vi "GET_Series.vi"(6 "get all issues":bool=TRUE, 7 "progress ref":refnum<vi>, 8 "error in (no error)":errorcluster, 10 "series URL":string, 11 "ComicVine_class in":refnum<class "series_class.lvclass">) -> (0 "error out":errorcluster, 3 "ComicVine_class out":refnum<class "series_class.lvclass">)   [LabVIEW 2024, in "series_class.lvclass"]
uses:
  series_class.lvclass
  series_class.lvclass/series_class.ctl
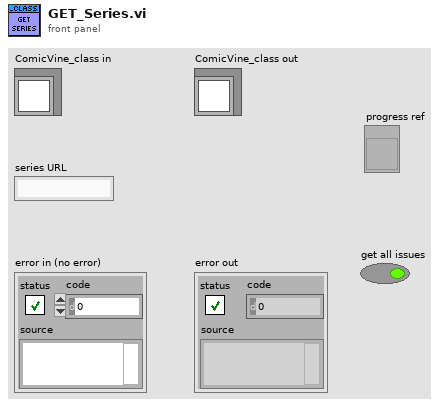
[diagram p1: front panel]
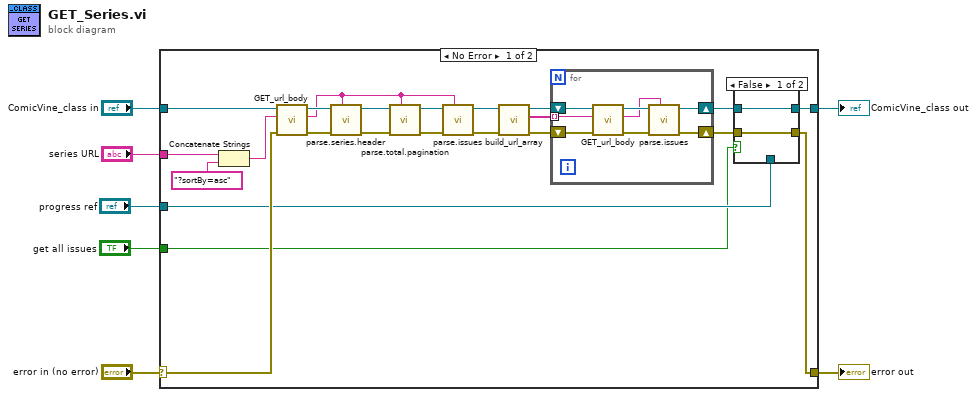
[diagram p0: block diagram]
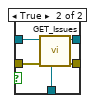
[diagram p2: hidden frame]
diagram:
  n1 = case shown="No Error" "error in (no error)" {
    selector: "error in (no error)" -> [w28 w47]
    tunnel: [w11 w47] -> w6
    tunnel: [w13 w46] -> w4
    tunnel: "ComicVine_class in" -> [w30 w46]
    tunnel: "series URL" -> [w23 _]
    tunnel: "progress ref" -> [w9 _]
    tunnel: "get all issues" -> [w8 _]
    frame No Error {
      n2 = Concatenate Strings(w23, "?sortBy=asc") -> (w22:string)
      n3 = call-dynamic "GET_url_body.vi"("error in (no error)"=w28, "url"=w22, "comic_class in"=w30) -> ("error out"=w27:errorcluster, "body"=w15:string, "comic_class out"=w29:refnum<class "series_class.lvclass">)  [unwired: 6 in]
      n4 = call "parse.series.header.vi"("series body"=w15, "error in (no error)"=w27, "ComicVine_class in"=w29) -> ("error out"=w25:errorcluster, "ComicVine_class out"=w26:refnum<class "series_class.lvclass">)  [unwired: 7 in]
      n5 = call "parse.total.pagination.vi"("series body"=w15, "error in (no error)"=w25, "ComicVine_class in"=w26) -> ("error out"=w10:errorcluster, "ComicVine_class out"=w21:refnum<class "series_class.lvclass">)  [unwired: 6 in, 1 out]
      n6 = call "parse.issues.vi"("series body"=w15, "error in (no error)"=w10, "ComicVine_class in"=w21) -> ("error out"=w19:errorcluster, "ComicVine_class out"=w20:refnum<class "series_class.lvclass">)  [unwired: 7 in]
      n7 = call "build_url_array.vi"("error in (no error)"=w19, "ComicVine_class in"=w20) -> ("error out"=w18:errorcluster, "urls"=w16:string[], "ComicVine_class out"=w17:refnum<class "series_class.lvclass">)  [unwired: 7 in]
      n8 = for {
        shift-right: [w39] -> w12
        shift-left: w18 -> [w42]
        shift-right: [w45] -> w14
        shift-left: w17 -> [w41]
        tunnel: w16 -> [w40] mode=indexing
        n9 = call-dynamic "GET_url_body.vi"("error in (no error)"=w42, "url"=w40, "comic_class in"=w41) -> ("error out"=w44:errorcluster, "body"=w38:string, "comic_class out"=w43:refnum<class "series_class.lvclass">)  [unwired: 6 in]
        n10 = call "parse.issues.vi"("series body"=w38, "error in (no error)"=w44, "ComicVine_class in"=w43) -> ("error out"=w39:errorcluster, "ComicVine_class out"=w45:refnum<class "series_class.lvclass">)  [unwired: 7 in]
      }
      n11 = case shown="False" w8 {
        tunnel: w14 -> [w31 w37]
        tunnel: [w31 w36] -> w13
        tunnel: w12 -> [w32 w35]
        tunnel: [w32 w34] -> w11
        tunnel: w9 -> [_ w33]
        frame False {
        }
        frame True {
          n12 = call "GET_Issues.vi"("progress ref"=w33, "error in (no error)"=w35, "series_class in"=w37) -> ("error out"=w34:errorcluster, "series_class out"=w36:refnum<class "series_class.lvclass">)  [unwired: 7 in]
        }
      }
    }
    frame Error {
    }
  }
  "error out" <- w6
  "ComicVine_class out" <- w4
